vi "Create G-CLI Script ClearCache.vi"(8 "error in (no error)":errorcluster, 11 "PostBuildSupport in":refnum<class "PostBuildSupport.lvclass">) -> (0 "error out":errorcluster, 2 "command":string, 3 "PostBuildSupport out":refnum<class "PostBuildSupport.lvclass">)   [LabVIEW 2019, in "PostBuildSupport.lvclass"]
uses:
  PostBuildSupport.lvclass
  PostBuildSupport.lvclass/PostBuildSupport.ctl
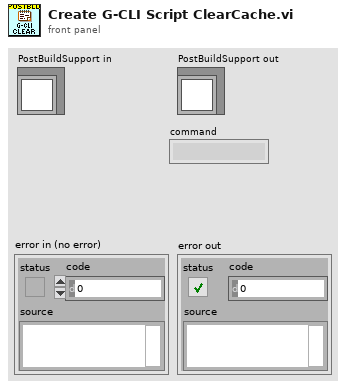
[diagram p1: front panel]
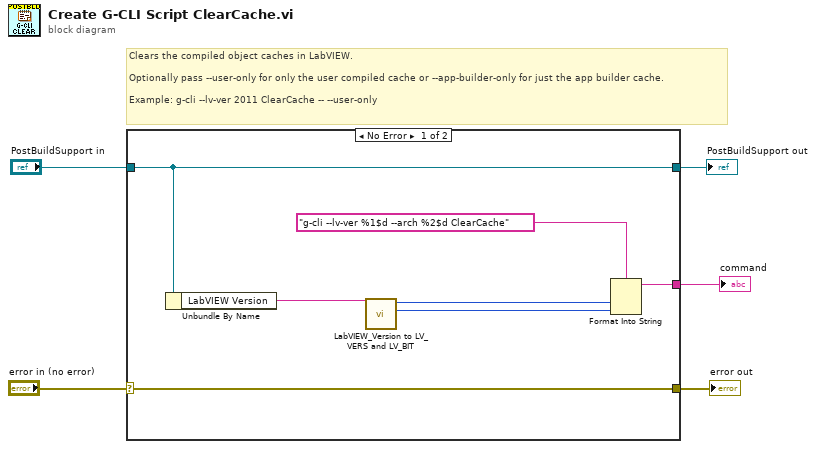
[diagram p0: block diagram]
diagram:
  # "Clears the compiled object caches in LabVIEW.\n\nOptionally pass --user-only for only the user compiled cache or --app-builder-only for just the app builder cache.\n\nExample: g-cli --lv-ver 2011 ClearCache -- --user-only"
  n1 = case shown="No Error" "error in (no error)" {
    selector: "error in (no error)" -> [w9 w14]
    tunnel: "PostBuildSupport in" -> [w12 w13]
    tunnel: [w9 w14] -> w3
    tunnel: [w12 w13] -> w2
    tunnel: [w10 _] -> w1
    frame No Error {
      n2 = Unbundle By Name(w12) -> ("LabVIEW Version"=w7:string)
      n3 = call "LabVIEW_Version to LV_VERS and LV_BIT.vi"("Package_LabVIEW_Version"=w7) -> ("LV_BIT"=w8:u32, "LV_VER"=w6:u32)  [unwired: 9 in]
      n4 = Format Into String(format string="g-cli --lv-ver %1$d --arch %2$d ClearCache", w6, w8) -> (resulting string=w10:string)  [unwired: 2 in, 1 out]
    }
    frame Error {
    }
  }
  "error out" <- w3
  "PostBuildSupport out" <- w2
  "command" <- w1
